vi "Save to file.vi"(10 "2D array":dbl[][](array[numeric]), 11 "File type":u16(ring) items=["Txt", "csv", "Excel"]) -> ()   [LabVIEW 2020]
doc: "This SubVi can save data from array to three diferrent kind of files"
uses:
  <vilib>/Utility/NIReport.llb/Report Type.ctl
  <vilib>/Utility/file.llb/Write Delimited Spreadsheet (string).vi
  <vilib>/addons/_office/excel.llb/Excel Easy Table (str).vi
  <vilib>/Utility/NIReport.llb/NI_report.lvclass
  <vilib>/Utility/NIReport.llb/NI_ReportGenerationCore.lvlib
  <vilib>/Utility/NIReport.llb/Excel/NI_Excel.lvclass
  <vilib>/addons/_office/NI_ReportGenerationToolkit.lvlib
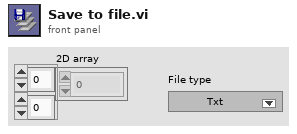
[diagram p1: front panel]
types:
  T1 = enum16{"open", "replace", "create", "open or create", "replace or create", "replace or create with confirmation"}
  T2 = typedef "NI_ReportGenerationCore.lvlib/Report Type.ctl" = enum16{"HTML", "Word", "Excel"}
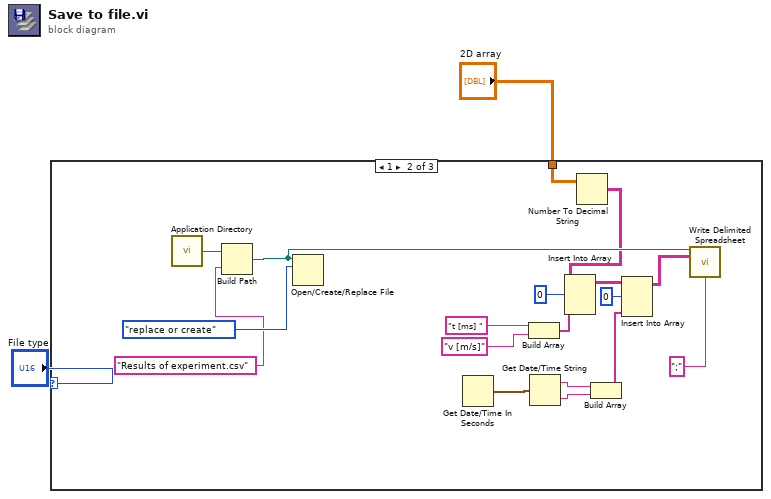
[diagram p0: block diagram]
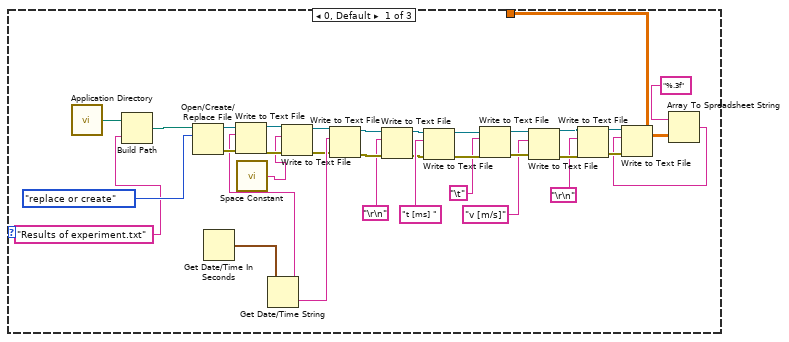
[diagram p2: hidden frame]
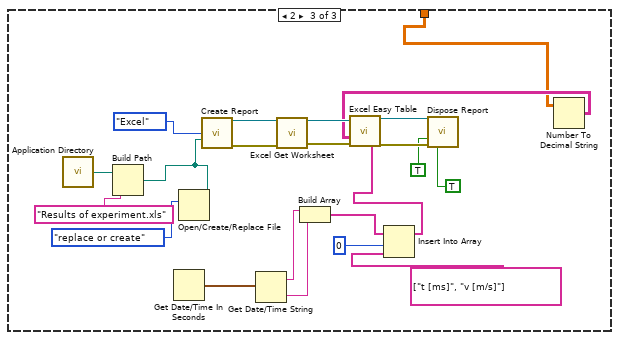
[diagram p3: hidden frame]
diagram:
  n1 = case shown="1" "File type" {
    tunnel: "2D array" -> [w18 w48 w61]
    frame 0, Default {
      n2 = call <vilib>:"Application Directory.vi"() -> ("Application Directory"=w26:path)
      n3 = Build Path(base path=w26, name or relative path="Results of experiment.txt") -> (appended path=w27:path)
      n4 = Open/Create/Replace File(file path (use dialog)=w27, operation (0:open)=T1."replace or create") -> (refnum out=w10:refnum<file>, error out=w5:errorcluster)  [unwired: 4 in, 1 out]
      n5 = Get Date/Time In Seconds() -> (seconds since 1Jan1904=w17:timestamp)
      n6 = call <vilib>:"Space Constant.vi"() -> ("String"=w3:string)
      n7 = Get Date/Time String(seconds (now)=w17) -> (date string=w4:string, time string=w16:string)  [unwired: 2 in]
      n8 = Write to Text File(file (use dialog)=w10, text=w4, error in=w5) -> (refnum out=w9:refnum<file>, error out=w6:errorcluster)  [unwired: 1 in, 1 out]
      n9 = Write to Text File(file (use dialog)=w9, text=w3, error in=w6) -> (refnum out=w8:refnum<file>, error out=w7:errorcluster)  [unwired: 1 in, 1 out]
      n10 = Write to Text File(file (use dialog)=w8, text=w16, error in=w7) -> (refnum out=w15:refnum<file>, error out=w12:errorcluster)  [unwired: 1 in, 1 out]
      n11 = Write to Text File(file (use dialog)=w15, text="\r\n", error in=w12) -> (refnum out=w14:refnum<file>, error out=w13:errorcluster)  [unwired: 1 in, 1 out]
      n12 = Write to Text File(file (use dialog)=w14, text="t [ms] ", error in=w13) -> (refnum out=w28:refnum<file>, error out=w33:errorcluster)  [unwired: 1 in, 1 out]
      n13 = Write to Text File(file (use dialog)=w28, text="\t", error in=w33) -> (refnum out=w29:refnum<file>, error out=w34:errorcluster)  [unwired: 1 in, 1 out]
      n14 = Write to Text File(file (use dialog)=w29, text="v [m/s]", error in=w34) -> (refnum out=w31:refnum<file>, error out=w35:errorcluster)  [unwired: 1 in, 1 out]
      n15 = Write to Text File(file (use dialog)=w31, text="\r\n", error in=w35) -> (refnum out=w32:refnum<file>, error out=w36:errorcluster)  [unwired: 1 in, 1 out]
      n16 = Array To Spreadsheet String(array=w18, 3:"%.3f" ("format string")) -> (spreadsheet string=w30:string)  [unwired: 1 in]
      n17 = Write to Text File(file (use dialog)=w32, text=w30, error in=w36) -> ()  [unwired: 1 in, 3 out]
    }
    frame 1 {
      n18 = call <vilib>:"Application Directory.vi"() -> ("Application Directory"=w54:path)
      n19 = Build Path(base path=w54, name or relative path="Results of experiment.csv") -> (appended path=w47:path)
      n20 = Open/Create/Replace File(file path (use dialog)=w47, operation (0:open)=T1."replace or create") -> ()  [unwired: 4 in, 3 out]
      n21 = Get Date/Time In Seconds() -> (seconds since 1Jan1904=w37:timestamp)
      n22 = Build Array("t [ms] " ("text"), "v [m/s]") -> (w45:string[])
      n23 = Get Date/Time String(seconds (now)=w37) -> (date string=w40:string, time string=w39:string)  [unwired: 2 in]
      n24 = Number To Decimal String(number=w48) -> (decimal integer string=w46:string[][])  [unwired: 1 in]
      n25 = Insert Into Array(array=w46, index (row)=0 ("index"), new element=w45) -> (w43:string[][])  [unwired: 1 in]
      n26 = Build Array(w40, w39) -> (w38:string[])
      n27 = Insert Into Array(array=w43, index (row)=0, new element=w38) -> (w42:string[][])  [unwired: 1 in]
      n28 = call-poly <vilib>:"Write Delimited Spreadsheet.vi"("file path (dialog if empty)"=w47, "2D data"=w42, "delimiter (\\t)"=";") -> ()  [unwired: 11 in, 2 out]
    }
    frame 2 {
      n29 = call <vilib>:"Application Directory.vi"() -> ("Application Directory"=w69:path)
      n30 = Build Path(base path=w69, name or relative path="Results of experiment.xls") -> (appended path=w70:path)
      n31 = Get Date/Time In Seconds() -> (seconds since 1Jan1904=w62:timestamp)
      n32 = Open/Create/Replace File(file path (use dialog)=w70, operation (0:open)=T1."replace or create") -> ()  [unwired: 4 in, 3 out]
      n33 = call <vilib>:"Create Report.vi"("report type"=Report_Type."Excel", "template (empty)"=w70) -> ("report out"=w71:refnum<class "NI_report.lvclass">, "error out"=w72:errorcluster)  [unwired: 12 in]
      n34 = Get Date/Time String(seconds (now)=w62) -> (date string=w60:string, time string=w59:string)  [unwired: 2 in]
      n35 = call <vilib>:"Excel Get Worksheet.vi"("report in"=w71, "error in (no error)"=w72) -> ("report out"=w73:refnum<class "NI_report.lvclass">, "error out"=w76:errorcluster)  [unwired: 12 in]
      n36 = Build Array(w60, w59) -> (w58:string[])
      n37 = Insert Into Array(array=w58, index=0, new element=string[] ["t [ms]", "v [m/s]"] ("column headers")) -> (w55:string[])
      n38 = Number To Decimal String(number=w61) -> (decimal integer string=w63:string[][])  [unwired: 1 in]
      n39 = call-poly <vilib>:"Excel Easy Table.vi"("report in"=w73, "text data"=w63, "error in (no error)"=w76, "column headers"=w55) -> ("report out"=w74:refnum<class "NI_report.lvclass">, "error out"=w75:errorcluster)  [unwired: 7 in, 3 out]
      n40 = call-dynamic "Dispose Report.vi"("report in"=w74, "save changes? (F)"=TRUE, "error in (no error)"=w75, "close report? (T)"=TRUE) -> ()  [unwired: 11 in, 1 out]
    }
  }
